vi "Get Data Name_csm.vi"(8 "error in (no error)":errorcluster, 11 "Data":variant) -> (0 "error out":errorcluster, 2 "Data Name":string, 3 "Data Dup":variant)   [LabVIEW 2017, in "Communicable State Machine.lvlib"]
doc: "Returns the name of the data wired on input."
uses:
  Communicable State Machine.lvlib
  <vilib>/Utility/Data Type/NI_Data Type.lvlib
panel:
  # "[OpenG VI Tags] ***Do Not Remove***"
  # "Get Data Name.vi\n\nReturns the name of the data wired on input.\n\nPlease visit http://www.OpenG.org to learn about the\nOpen Source LabVIEW software movement.\n\nNOTICE -- YOU MUST LEAVE THIS NOTICE IN PLACE.  PER THE TERMS OF THE LICENSE BELOW, YOU MAY SUBLICENSE THIS SOFTWARE \nIN ANY WAY THAT DOES NOT CONFLICT WITH THIS LICENSE.\n\n### BSD License (http://www.opensource.org/licenses/bsd-license.php) Begin ###\n \nCopyright (c) 2002, Jean-Pierre Drolet <drolet_jp@hotmail.com>\nCopyright (c) 2002-2006, Jim Kring <jim@jimkring.com>\n\nAll rights reserved.\n\nRedistribution and use in source and binary forms, with or without modification, are permitted provided that the following conditions are met:\n\n    * Redistributions of source code must retain the above copyright notice, this list of conditions and the following disclaimer.\n    * Redistributions in binary form must reproduce the above copyright notice, this list of conditions and the following disclaimer in the \n       documentation and/or other materials provided with the distribution.\n    * Neither the name of SciWare, James Kring, Inc., nor the names of its contributors may be used to endorse or promote products derived \n       from this software without specific prior written permission.\n\nTHIS SOFTWARE IS PROVIDED BY THE COPYRIGHT HOLDERS AND CONTRIBUTORS \"AS IS\" AND ANY EXPRESS OR IMPLIED WARRANTIES, \nINCLUDING, BUT NOT LIMITED TO, THE IMPLIED WARRANTIES OF MERCHANTABILITY AND FITNESS FOR A PARTICULAR PURPOSE ARE \nDISCLAIMED. IN NO EVENT SHALL THE COPYRIGHT OWNER OR CONTRIBUTORS BE LIABLE FOR ANY DIRECT, INDIRECT, INCIDENTAL,\n SPECIAL, EXEMPLARY, OR CONSEQUENTIAL DAMAGES (INCLUDING, BUT NOT LIMITED TO, PROCUREMENT OF SUBSTITUTE GOODS OR \nSERVICES; LOSS OF USE, DATA, OR PROFITS; OR BUSINESS INTERRUPTION) HOWEVER CAUSED AND ON ANY THEORY OF LIABILITY, \nWHETHER IN CONTRACT, STRICT LIABILITY, OR TORT (INCLUDING NEGLIGENCE OR OTHERWISE) ARISING IN ANY WAY OUT OF THE USE \nOF THIS SOFTWARE, EVEN IF ADVISED OF THE POSSIBILITY OF SUCH DAMAGE.\n\n### BSD License End ###"
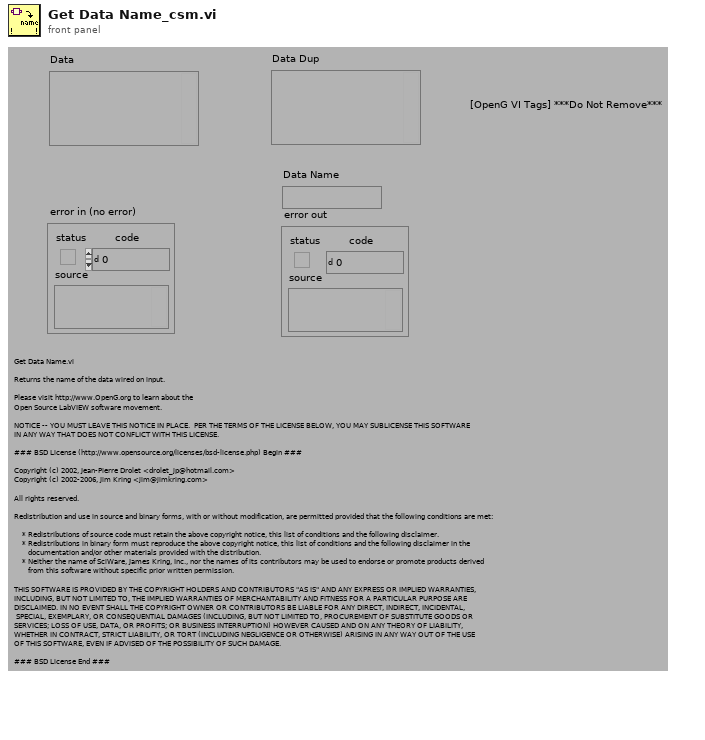
[diagram p1: front panel]
types:
  T1 = cluster{"length":u16, "private":u8, "type":enum8{"<Null>", "I8", "I16", "I32", "I64", "U8", "U16", "U32", "U64", "SGL", "DBL", "EXT", "CSG", "CDB", "CXT", "0x0F", "0x10", "0x11", "0x12", "0x13", "0x14", "Enum U8", "Enum U16", "Enum U32", "Enum U64", "SGL PQ", "DBL PQ", "EXT PQ", "CSG PQ", "CDB PQ", "CXT PQ", "0x1F", "0x20", "Boolean", "0x22", "0x23", "0x24", "0x25", "0x26", "0x27", "0x28", "0x29", "0x2A", "0x2B", "0x2C", "0x2D", "0x2E", "0x2F", "String", "0x31", "Path", "Pict", "0x34", "0x35", "0x36", "DAQ", "0x38", "0x39", "0x3A", "0x3B", "0x3C", "0x3D", "0x3E", "0x3F", "Array", "0x41", "0x42", "0x43", "0x44", "0x45", "0x46", "0x47", "0x48", "0x49", "0x4A", "0x4B", "0x4C", "0x4D", "0x4E", "0x4F", "Cluster", "0x51", "0x52", "Variant", "Waveform", "0x55", "0x56", "0x57", "0x58", "0x59", "0x5A", "0x5B", "0x5C", "0x5D", "0x5E", "Fixed Point", "0x60", "0x61", "0x62", "0x63", "0x64", "0x65", "0x66", "0x67", "0x68", "0x69", "0x6A", "0x6B", "0x6C", "0x6D", "0x6E", "0x6F", "Refnum", "0x71", "0x72", "Set Collection", "Map Collection"}, "# elements":u16}
  T2 = enum8{"<Null>", "I8", "I16", "I32", "I64", "U8", "U16", "U32", "U64", "SGL", "DBL", "EXT", "CSG", "CDB", "CXT", "0x0F", "0x10", "0x11", "0x12", "0x13", "0x14", "Enum U8", "Enum U16", "Enum U32", "Enum U64", "SGL PQ", "DBL PQ", "EXT PQ", "CSG PQ", "CDB PQ", "CXT PQ", "0x1F", "0x20", "Boolean", "0x22", "0x23", "0x24", "0x25", "0x26", "0x27", "0x28", "0x29", "0x2A", "0x2B", "0x2C", "0x2D", "0x2E", "0x2F", "String", "0x31", "Path", "Pict", "0x34", "0x35", "0x36", "DAQ", "0x38", "0x39", "0x3A", "0x3B", "0x3C", "0x3D", "0x3E", "0x3F", "Array", "0x41", "0x42", "0x43", "0x44", "0x45", "0x46", "0x47", "0x48", "0x49", "0x4A", "0x4B", "0x4C", "0x4D", "0x4E", "0x4F", "Cluster", "0x51", "0x52", "Variant", "Waveform", "0x55", "0x56", "0x57", "0x58", "0x59", "0x5A", "0x5B", "0x5C", "0x5D", "0x5E", "Fixed Point", "0x60", "0x61", "0x62", "0x63", "0x64", "0x65", "0x66", "0x67", "0x68", "0x69", "0x6A", "0x6B", "0x6C", "0x6D", "0x6E", "0x6F", "Refnum", "0x71", "0x72", "Set Collection", "Map Collection"}
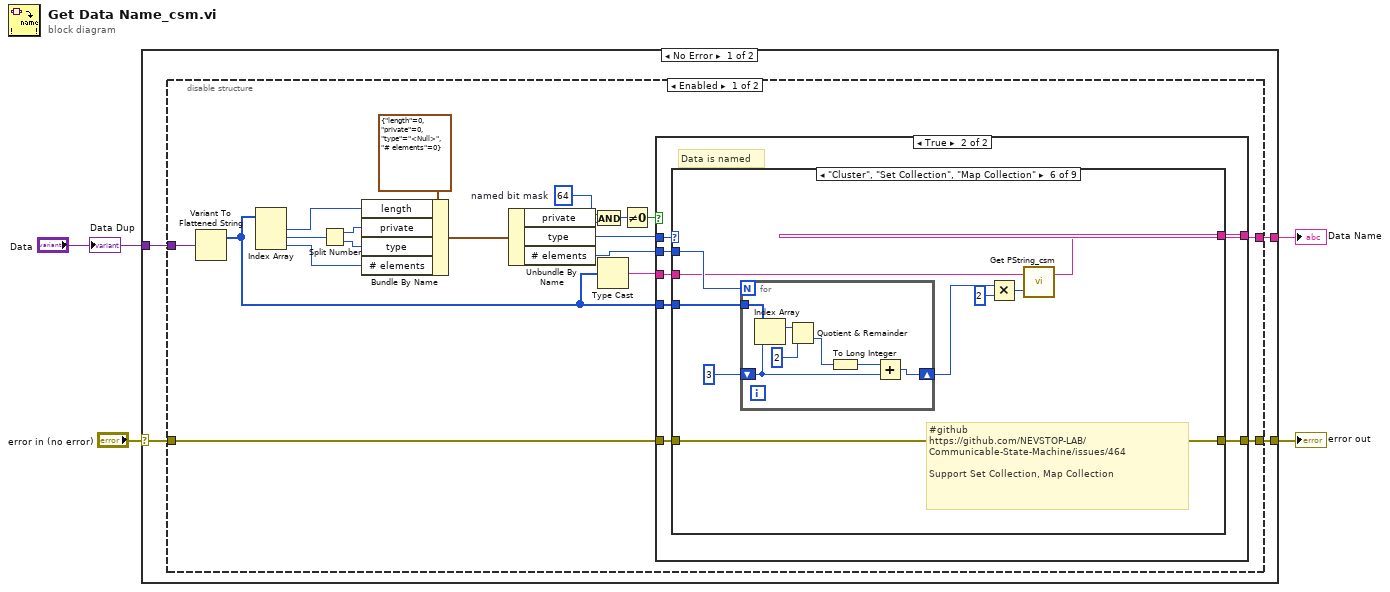
[diagram p0: block diagram]
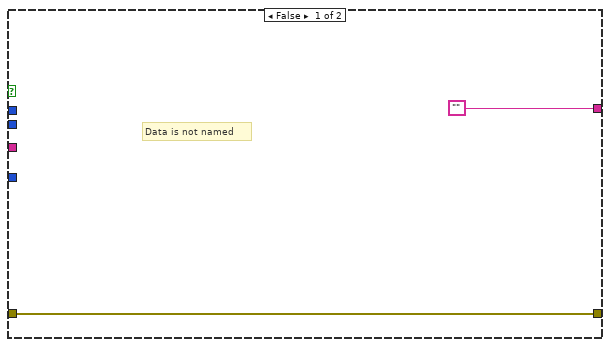
[diagram p2: hidden frame]
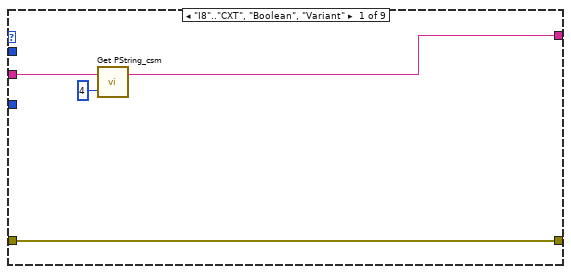
[diagram p3: hidden frame]
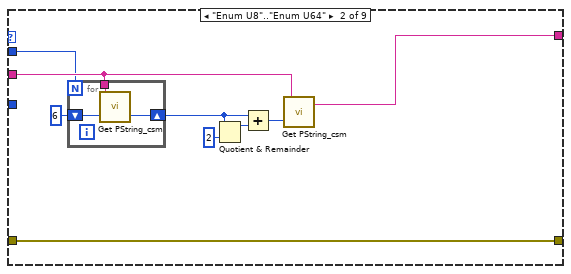
[diagram p4: hidden frame]
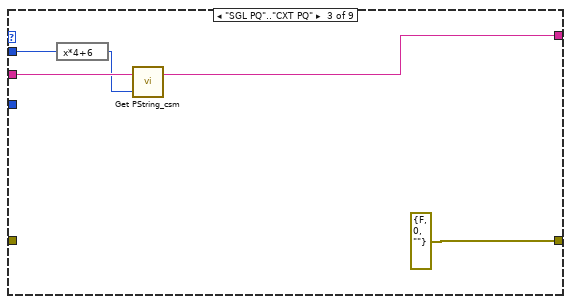
[diagram p5: hidden frame]
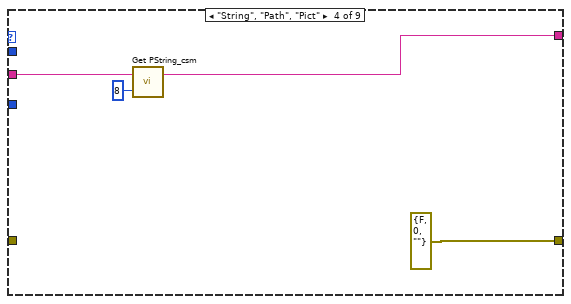
[diagram p6: hidden frame]
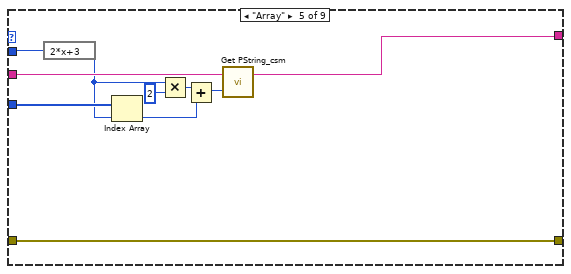
[diagram p7: hidden frame]
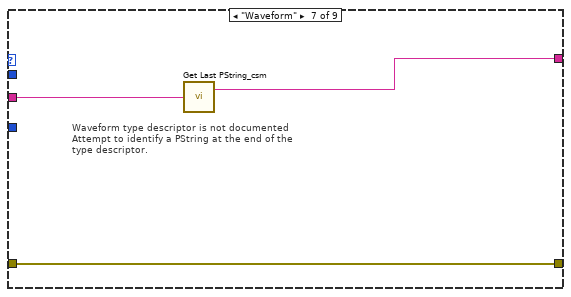
[diagram p8: hidden frame]
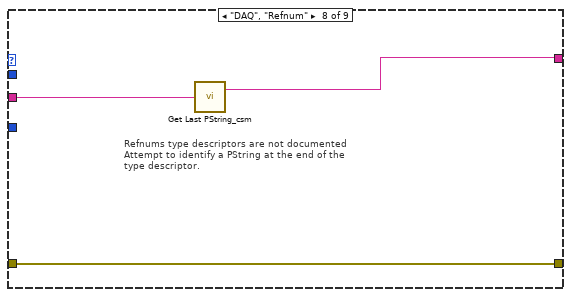
[diagram p9: hidden frame]
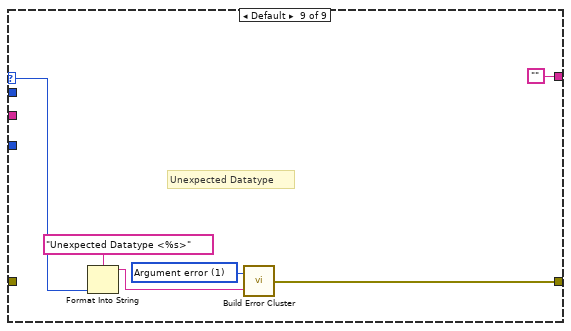
[diagram p10: hidden frame]
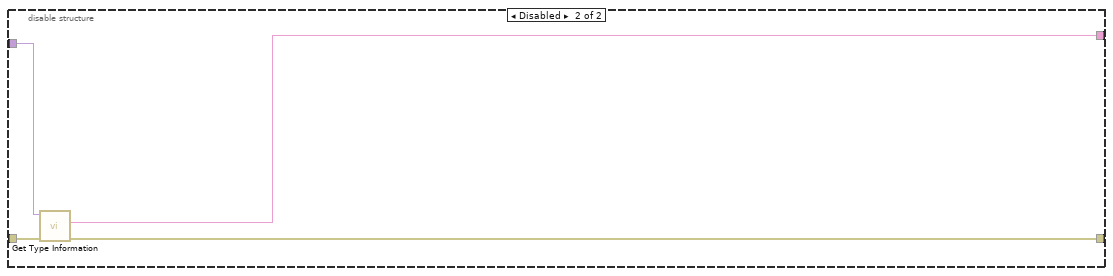
[diagram p11: hidden frame]
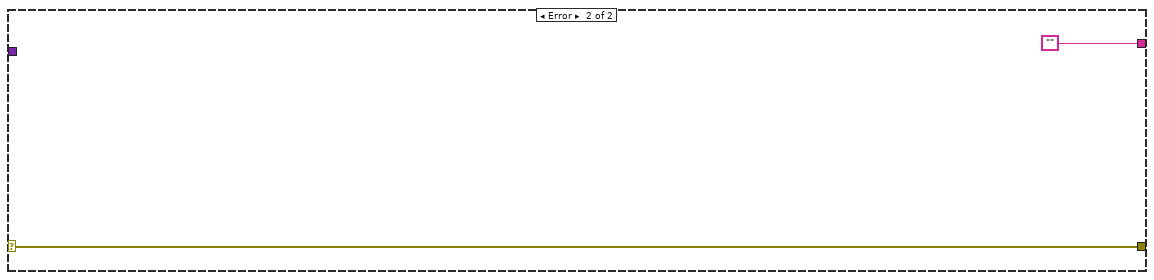
[diagram p12: hidden frame]
diagram:
  n1 = case shown="No Error" "error in (no error)" {
    selector: "error in (no error)" -> [w5 w105]
    tunnel: [w8 w105] -> w4
    tunnel: [w7 ""] -> w2
    tunnel: "Data" -> [w6 _]
    frame No Error {
      n2 = disable-structure shown="Enabled" {
        disable-tunnel: [w27 w101] -> w8
        disable-tunnel: [w26 w100] -> w7
        disable-tunnel: w6 -> [w25 w102]
        disable-tunnel: w5 -> [w15 w103]
        frame Enabled {
          w18 = u8 64  # named bit mask
          n3 = Variant To Flattened String(Variant=w25) -> (1:w24:i16[])  [unwired: 1 out]
          n4 = Index Array(array=w24) -> (element #1=w10:i16, element #2=w13:i16, element #3=w14:i16)  [unwired: 3 in]
          n5 = Split Number(x=w13) -> (hi(x)=w11:u8, lo(x)=w12:u8)
          n6 = Bundle By Name(cluster=T1 {"length"=0, "private"=0, "type"=enum."<Null>", "# elements"=0} ("Type Descriptor Header"), "length"=w10, "private"=w11, "type"=w12, "# elements"=w14) -> (w23:T1)
          n7 = Unbundle By Name(w23) -> ("private"=w17:u8, "type"=w16:T2, "# elements"=w22:u16)
          n8 = And(x=w18, y=w17) -> (x .and. y?=w20:u8)
          n9 = Type Cast(x=w24) -> (*(type *) &x=w21:string)  [unwired: 1 in]
          n10 = Not Equal To 0?(x=w20) -> (x != 0?=w19:bool)
          n11 = case shown="True" w19 {
            tunnel: [w28 w36] -> w27
            tunnel: w16 -> [_ w35]
            tunnel: w21 -> [_ w34]
            tunnel: ["" w33] -> w26
            tunnel: w22 -> [_ w32]
            tunnel: w24 -> [_ w31]
            tunnel: w15 -> [w28 w30]
            frame False {
              # "Data is not named"
            }
            frame True {
              # "Data is named"
              n12 = case shown="\"Cluster\", \"Set Collection\", \"Map Collection\"" w35 {
                selector: w35 -> [_ _ _ _ _ _ _ _ w94]
                tunnel: [w37 w41 errorcluster {"status"=FALSE, "code"=0, "source"=""} ("error out") errorcluster {"status"=FALSE, "code"=0, "source"=""} ("error out") w62 w72 w88 w91 w99] -> w36
                tunnel: w34 -> [w40 w46 w56 w61 w69 w78 w90 w93 _]
                tunnel: [w38 w45 w54 w60 w68 w77 w89 w92 ""] -> w33
                tunnel: w32 -> [_ w44 w57 _ w71 w80 _ _ _]
                tunnel: w31 -> [_ _ _ _ w70 w79 _ _ _]
                tunnel: w30 -> [w37 w41 _ _ w62 w72 w88 w91 _]
                frame "I8".."CXT", "Boolean", "Variant" {
                  n13 = call "Get PString_csm.vi"("Offset (0)"=4 ("offset (0)"), "String"=w40) -> ("PString"=w38:string)  [unwired: 1 out]
                }
                frame "Enum U8".."Enum U64" {
                  n14 = for {
                    N: w44 -> [_]
                    tunnel: w46 -> [w50]
                    shift-right: [w51] -> w48
                    shift-left: 6 -> [w52]
                    n15 = call "Get PString_csm.vi"("Offset (0)"=w52, "String"=w50) -> ("Offset Past PString"=w51:i32)  [unwired: 1 out]
                  }
                  n16 = Quotient & Remainder(x=w48, y=2) -> (x-y*floor(x/y)=w42:i32)  [unwired: 1 out]
                  n17 = Add(x=w48, y=w42) -> (x+y=w47:i32)
                  n18 = call "Get PString_csm.vi"("Offset (0)"=w47, "String"=w46) -> ("PString"=w45:string)  [unwired: 1 out]
                }
                frame "SGL PQ".."CXT PQ" {
                  n19 = expression code="x*4+6"(w57) -> (w55:u16)
                  n20 = call "Get PString_csm.vi"("Offset (0)"=w55, "String"=w56) -> ("PString"=w54:string)  [unwired: 1 out]
                }
                frame "String", "Path", "Pict" {
                  n21 = call "Get PString_csm.vi"("Offset (0)"=8 ("offset (0)"), "String"=w61) -> ("PString"=w60:string)  [unwired: 1 out]
                }
                frame "Array" {
                  n22 = expression code="2*x+3"(w71) -> (w67:u16)
                  n23 = Index Array(array=w70, index=w67) -> (element=w64:i16)
                  n24 = Multiply(x=w67, y=u16 2) -> (x*y=w65:u16)
                  n25 = Add(x=w65, y=w64) -> (x+y=w63:u16)
                  n26 = call "Get PString_csm.vi"("Offset (0)"=w63, "String"=w69) -> ("PString"=w68:string)  [unwired: 1 out]
                }
                frame "Cluster", "Set Collection", "Map Collection" {
                  # "#github \nhttps://github.com/NEVSTOP-LAB/Communicable-State-Machine/issues/464\n\nSupport Set Collection, Map Collection"
                  n27 = for {
                    N: w80 -> [_]
                    shift-right: [w86] -> w75
                    shift-left: 3 -> [w85]
                    tunnel: w79 -> [w87]
                    n28 = Index Array(array=w87, index=w85) -> (element=w83:i16)
                    n29 = Quotient & Remainder(x=w83, y=i16 2) -> (floor(x/y)=w84:i16)  [unwired: 1 out]
                    n30 = To Long Integer(number=w84) -> (32bit integer=w81:i32)
                    n31 = Add(x=w81, y=w85) -> (x+y=w86:i32)
                  }
                  n32 = Multiply(x=w75, y=2) -> (x*y=w74:i32)
                  n33 = call "Get PString_csm.vi"("Offset (0)"=w74, "String"=w78) -> ("PString"=w77:string)  [unwired: 1 out]
                }
                frame "Waveform" {
                  # "Waveform type descriptor is not documented\nAttempt to identify a PString at the end of the\ntype descriptor."
                  n34 = call "Get Last PString_csm.vi"("String"=w90) -> ("Last PString"=w89:string)  [unwired: 1 out]
                }
                frame "DAQ", "Refnum" {
                  # "Refnums type descriptors are not documented\nAttempt to identify a PString at the end of the\ntype descriptor."
                  n35 = call "Get Last PString_csm.vi"("String"=w93) -> ("Last PString"=w92:string)  [unwired: 1 out]
                }
                frame Default {
                  w98 = 1 items=["No error", "Argument error", "Memory is full", "Out of zone", "End of file", "File already open", "Generic file I/O error", "File not found", "File permission error", "Disk is full", "Duplicate path", "Too many files open", "System feature not enabled", "Resource file not found", "Cannot add resource", "Resource not found", "Image not found", "Image memory error", "Pen does not exist", "Config type invalid", "Config token not found", "Config parse error", "Config memory error", "Bad external code format", "Bad external code offset", "External code not present", "Null window", "Destroy window error", "Null menu", "Print aborted", "Bad print record", "Print driver error", "Windows error during printing", "Memory error during printing", "Print dialog error", "Generic print error", "Invalid device refnum", "Device not found", "Device parameter error", "Device unit error", "Cannot open device", "Device call aborted", "Generic error", "Cancelled by user", "Object ID too low", "Object ID too high", "Object not in heap", "Unknown heap", "Unknown object (invalid DefProc)", "Unknown object (DefProc not in table)", "Message out of range", "Invalid (null) method", "Unknown message", "Manager call not supported", "Bad address", "Network operation in progress", "Network operation timed out", "Connection is busy", "Network attribute not supported", "Network error", "Address in use", "System out of memory", "Connection aborted", "Connection refused", "Not connected", "Already connected", "Connection closed", "Initialization error (interapplication manager)", "Bad occurrence", "Wait on unbound occurrence handler", "Occurrence queue overflow", "Datalog type conflict", "Unused", "Unrecognized type (interapplication manager)", "Memory corrupt", "Failed to make temporary DLL", "Old CIN version", "Drag socket not found", "Failed to load drop-object", "Failed to register OLE object", "Failed to release OLE object", "Format specifier type mismatch", "Unknown format specifier", "Too few format specifiers", "Too many format specifiers", "Scan failed", "Newer CIN version", "Error converting to variant", "Runtime menu error", "Password tampered", "Variant attribute not found", "Incompatible variant data type", "Event data is not available", "Event Store is not present", "Occurrence is not found", "Event Queue is not created", "Event info is not available", "Refnum passed is NULL", "Error retrieving Class GUID", "Error retrieving CoClass GUID", "Error retrieving TypeLib GUID.", "Bad built application magic bytes.", "Specific driver is different from the specific driver associated with the Logical Name.", "There is no session opened to the class driver.", "Max Error", "MAX - Error with config objects", "MAX - Error loading configuration", "MAX - Group not supported"]
                  # "Unexpected Datatype"
                  n36 = Format Into String(format string="Unexpected Datatype <%s>" ("Format String"), w94) -> (resulting string=w95:string)  [unwired: 2 in, 1 out]
                  n37 = call "Build Error Cluster.vi"("String to Prepend to Source (\"\")"=w95, "Code"=w98) -> ("error out"=w99:errorcluster)
                }
              }
            }
          }
        }
        frame Disabled {
          n38 = call <vilib>:"Get Type Information.vi"("error in (no error)"=w103, "Variant"=w102) -> ("error out"=w101:errorcluster, "Name"=w100:string)  [unwired: 5 in, 3 out]
        }
      }
    }
    frame Error {
    }
  }
  "error out" <- w4
  "Data Name" <- w2
  "Data Dup" <- "Data"
